vi "Parameter Set Read Single.vi"(8 "error in":errorcluster, 9 "Channel Index":i32, 11 "Parameter Set in":refnum<class "Parameter Set.lvclass">) -> (0 "error out":errorcluster, 1 "Changed or First Call?":bool, 2 "Parameter Set CTL":i32, 3 "Parameter Set out":refnum<class "Parameter Set.lvclass">)   [LabVIEW 2023, in "Parameter Set.lvclass"]
uses:
  Parameter Set.lvclass
  Parameter Set.lvclass/Parameter Set.ctl
  <vilib>/ADAS Replay HIL/Channels/Tag Wrapper/Polymorphic/Read Channel (I32).vi
  a75b5895-1da4-4397-9b19-9a359f0c58bf.vi
  <vilib>/ADAS Replay HIL/Channels/Tag Wrapper/Polymorphic/Read Channel (I32).vi/b2f764de-0c1e-4784-a155-687fc995a684.vi
  <vilib>/ADAS Replay HIL/Channels/Tag Wrapper/Polymorphic/Read Channel (I32).vi/b2f764de-0c1e-4784-a155-687fc995a684.vi/c28b0ead-42ad-4072-80a2-aca7f2bd7ce3.vi
  <vilib>/ADAS Replay HIL/Channels/Tag Wrapper/Polymorphic/Read Channel (I32).vi/b2f764de-0c1e-4784-a155-687fc995a684.vi/219d0231-d98b-4193-b5cc-84f90e3c9091.vi
  <vilib>/ADAS Replay HIL/Channels/Tag Wrapper/Tag Wrapper.lvlib
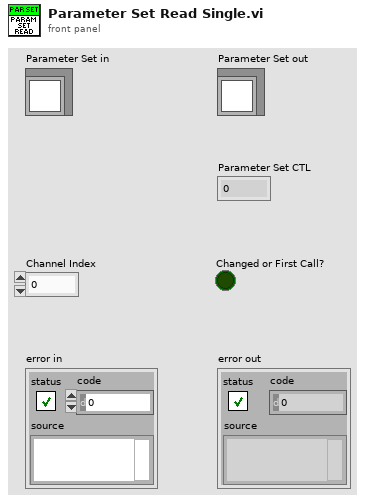
[diagram p1: front panel]
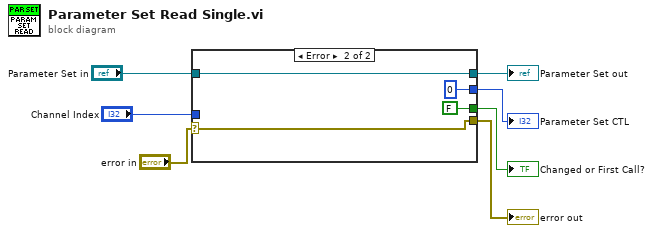
[diagram p0: block diagram]
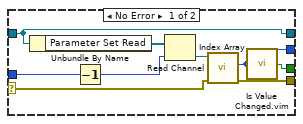
[diagram p2: hidden frame]
diagram:
  n1 = case shown="Error" "error in" {
    selector: "error in" -> [w11 w20]
    tunnel: [w10 w20] -> w6
    tunnel: [w13 w19] -> w4
    tunnel: "Parameter Set in" -> [w13 w19]
    tunnel: "Channel Index" -> [w12 _]
    tunnel: [w9 0 ("Value out")] -> w2
    tunnel: [w8 FALSE ("changed or first call?")] -> w1
    frame No Error {
      n2 = Unbundle By Name(w13) -> ("Parameter Set Read"=w16:refnum<k21>[])
      n3 = Decrement(x=w12) -> (x-1=w15:i32)
      n4 = Index Array(array=w16, index=w15) -> (element=w14:refnum<k21>)
      n5 = call-poly <vilib>:"Read Channel.vi"("error in"=w11, "ADAS HIL Channel in"=w14) -> ("error out"=w10:errorcluster, "Value out"=w9:i32)  [unwired: 6 in, 2 out]
      n6 = call "Is Value Changed.vim"("value"=w9) -> ("changed or first call?"=w8:bool)
    }
    frame Error {
    }
  }
  "error out" <- w6
  "Parameter Set out" <- w4
  "Parameter Set CTL" <- w2
  "Changed or First Call?" <- w1
